vi "Open CSM_Tool_Launcher.vi"() -> ()   [LabVIEW 2017, in "csm_tool_menu.lvlib"]
uses:
  csm_tool_menu.lvlib
  fd0165b5-6fc4-4d2a-af44-7735b0eff26e.vi
  user.lib/_NEVSTOP/Communicable State Machine(CSM)/_xnode/csm_tool/_xnode_csm_tool_support/CSM DebugTool Dialog.lvlib
  user.lib/_NEVSTOP/Communicable State Machine(CSM)/_tool/_ui/csm-ui-support.lvlib
panel:
  in  "error in (no error)":errorcluster
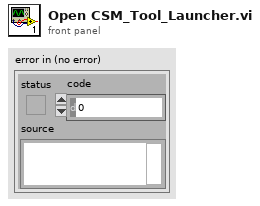
[diagram p1: front panel]
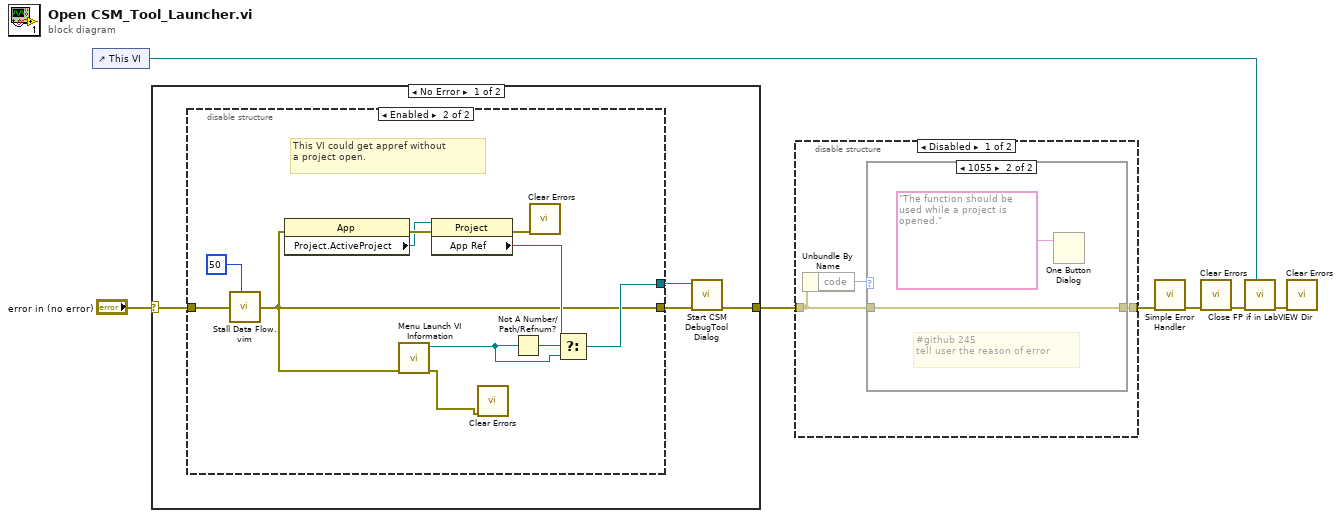
[diagram p0: block diagram]
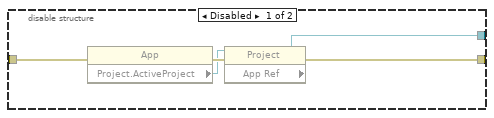
[diagram p2: hidden frame]
diagram:
  n1 = control-ref of="This VI"() -> (w4:refnum<vi>)
  n2 = case shown="No Error" "error in (no error)" {
    selector: "error in (no error)" -> [w11 w28]
    tunnel: [w8 w28] -> w2
    frame No Error {
      n3 = disable-structure shown="Enabled" {
        disable-tunnel: w11 -> [w16 w21]
        disable-tunnel: [w13 w18] -> w10
        disable-tunnel: [w12 w22] -> w9
        frame Disabled {
          n4 = property class="App"(error in=w16) -> (error out=w15:errorcluster, "Project.ActiveProject"=w14:refnum<vi>)  [unwired: 1 in, 1 out]
          n5 = property class="Project"(reference=w14, error in=w15) -> (error out=w13:errorcluster, "App Ref"=w12:refnum<vi>)  [unwired: 1 out]
        }
        frame Enabled {
          # "This VI could get appref without \na project open."
          n6 = call "Stall Data Flow.vim"("value in"=w21, "milliseconds to wait"=u32 50) -> ("value out"=w18:errorcluster)  [unwired: 1 out]
          n7 = property class="App"(error in=w18) -> (error out=w26:errorcluster, "Project.ActiveProject"=w25:refnum<vi>)  [unwired: 1 in, 1 out]
          n8 = call <vilib>:"Menu Launch VI Information.vi"("error in (no error)"=w18) -> ("error out"=w19:errorcluster, "Menu Launch:App"=w24:refnum<vi>)  [unwired: 8 in, 1 out]
          n9 = property class="Project"(reference=w25, error in=w26) -> (error out=w20:errorcluster, "App Ref"=w23:refnum<vi>)  [unwired: 1 out]
          n10 = call <vilib>:"Clear Errors.vi"("error in (no error)"=w19) -> ()  [unwired: 5 in, 2 out]
          n11 = Not A Number/Path/Refnum?(number/path/refnum=w24) -> (NaN/Path/Refnum?=w27:bool)
          n12 = call <vilib>:"Clear Errors.vi"("error in (no error)"=w20) -> ()  [unwired: 5 in, 2 out]
          n13 = Select(t=w23, s=w27, f=w24) -> (s? t:f=w22:refnum<vi>)
        }
      }
      n14 = call "Start CSM DebugTool Dialog.vi"("error in (no error)"=w10, "Application In"=w9) -> ("error out"=w8:errorcluster)  [unwired: 9 in]
    }
    frame Error {
    }
  }
  n15 = disable-structure shown="Disabled" {
    disable-tunnel: [w31 w35] -> w3
    disable-tunnel: w2 -> [w30 w35]
    frame Disabled {
      n16 = Unbundle By Name(w30) -> ("code"=w29:i32)
      n17 = case shown="1055" w29 {
        tunnel: w30 -> [w32 w34]
        tunnel: [w32 w34] -> w31
        frame 0, Default {
        }
        frame 1055 {
          # "#github 245\ntell user the reason of error"
          n18 = One Button Dialog(message="The function should be used while a project is opened.") -> ()  [unwired: 1 in, 1 out]
        }
      }
    }
    frame Enabled {
    }
  }
  n19 = call <vilib>:"Simple Error Handler.vi"("error in (no error)"=w3) -> ("error out"=w1:errorcluster)  [unwired: 4 in, 4 out]
  n20 = call <vilib>:"Clear Errors.vi"("error in (no error)"=w1) -> ("error out"=w6:errorcluster)  [unwired: 5 in, 1 out]
  n21 = call "Close FP if in LabVIEW Dir.vi"("VI Refnum"=w4, "Error in"=w6) -> ("Error out"=w7:errorcluster)  [unwired: 9 in]
  n22 = call <vilib>:"Clear Errors.vi"("error in (no error)"=w7) -> ()  [unwired: 5 in, 2 out]
